vi "LSX Set BPZ Joyspeed.vi"(8 "error in (no error)":errorcluster, 9 "dAValue":dbl, 10 "lAPar":i32, 11 "lLSID":i32) -> (0 "error out":errorcluster, 3 "function return":i32)   [LabVIEW 2018, in "Tango.lvlib"]
doc: "TANGOAPI int TANGOCALL LSX_SetBPZJoyspeed (int lLSID, int lAPar, double dAValue);"
uses:
  Tango.lvlib
  SubVIs/Tango_DLL.dll
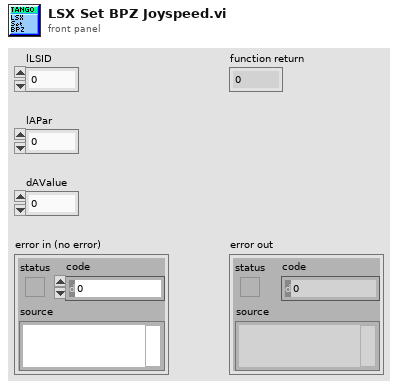
[diagram p1: front panel]
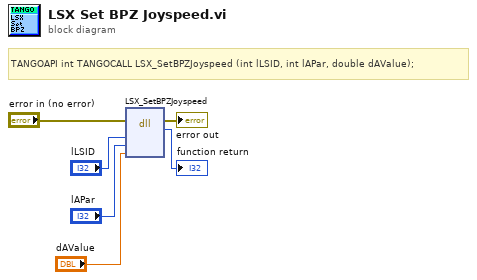
[diagram p0: block diagram]
diagram:
  # "TANGOAPI int TANGOCALL LSX_SetBPZJoyspeed (int lLSID, int lAPar, double dAValue);"
  n1 = dll-call lib="C:/Users/Familie/Documents/LabviewIX81/lib/TANGO Stage/SubVIs/Tango_DLL.*" fn="LSX_SetBPZJoyspeed"(error in="error in (no error)", "lLSID"="lLSID", "lAPar"="lAPar", "dAValue"="dAValue") -> (error out=→"error out":errorcluster, →"function return":i32)  [unwired: 5 in, 1 out]
